vi "saveBackgroundMedian.vi"() -> ()   [LabVIEW 2012]
uses:
  <vilib>/userdefined/High Color/IMAQdx.ctl
  <vilib>/vision/driver/NI_Vision_Acquisition_Software.lvlib
  <vilib>/vision/NI_Vision_Development_Module.lvlib
  <resource>/objmgr/IMAQImage.rc
panel:
  out "element 2":i32
  out "element":i32
  out "Array":u8[][][](array[numeric])
  in  "Camera Name":T1
  out "Image Array":T2[](array[plugin-control])
  in  "Number of Images":i32=5
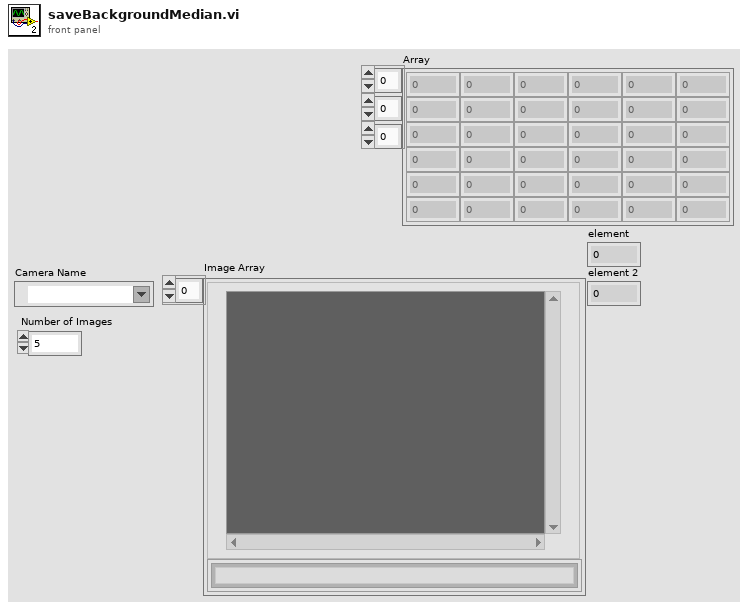
[diagram p1: front panel]
types:
  T1 = typedef "IMAQdx.ctl" = refnum<k21>
  T2 = typedef "IMAQ Image.ctl" = refnum<image>
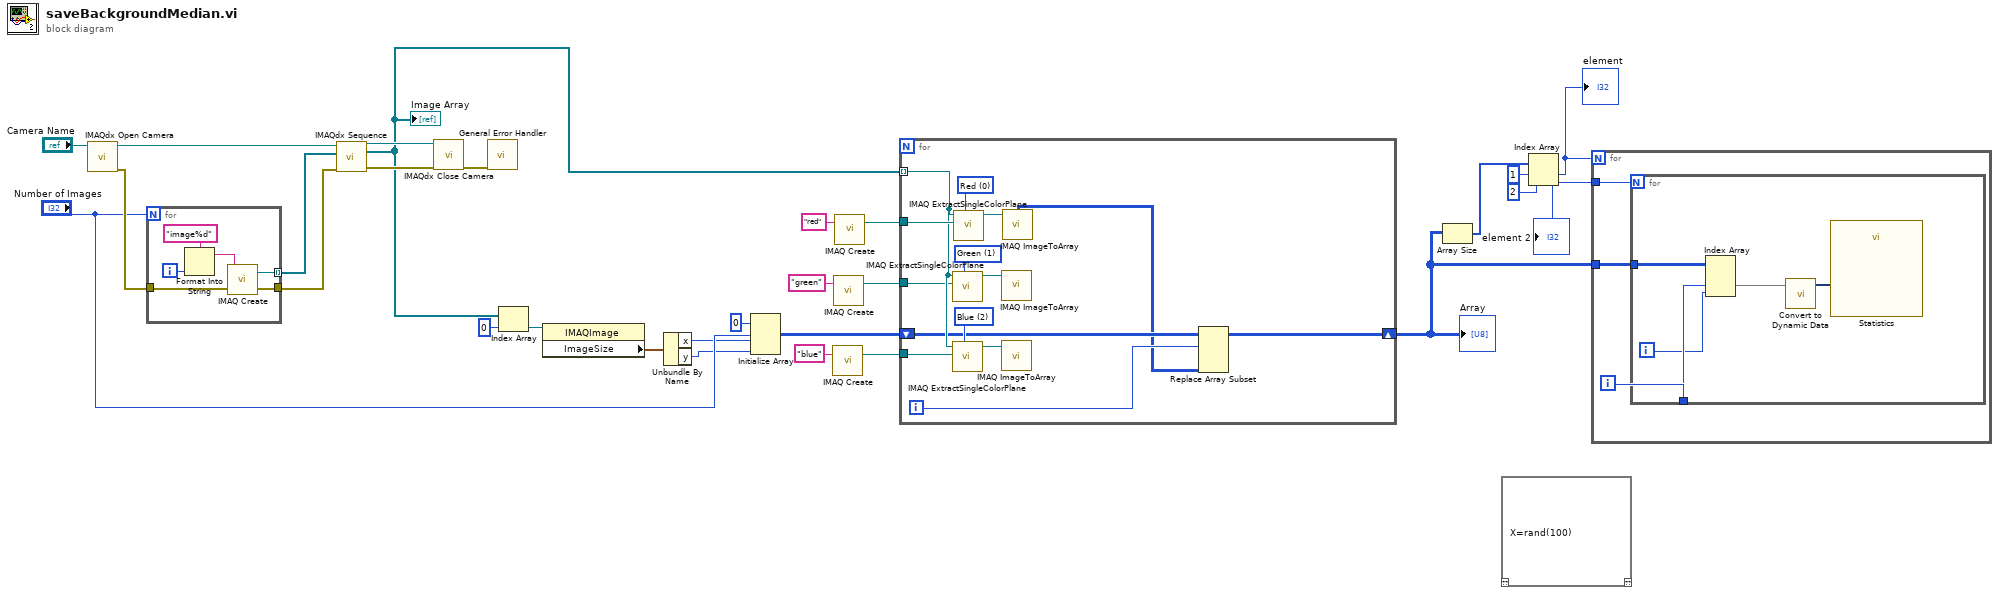
[diagram p0: block diagram]
diagram:
  n1 = call <vilib>:"IMAQdx Open Camera.vi"("Session In"="Camera Name") -> ("error out"=w27:errorcluster, "Session Out"=w23:T1)  [unwired: 2 in, 7 out]
  n2 = for {
    N: "Number of Images" -> [_]
    tunnel: w27 -> [w35]
    tunnel: [w34] -> w25 mode=indexing
    tunnel: [w33] -> w26
    i -> [w32]
    n3 = Format Into String(format string="image%d" ("Image Name"), w32) -> (resulting string=w31:string)  [unwired: 2 in, 1 out]
    n4 = call "IMAQ Create"("Image Name"=w31, "error in (no error)"=w35) -> ("New Image"=w34:T2, "error out"=w33:errorcluster)  [unwired: 2 in, 1 out]
  }
  n5 = call <vilib>:"IMAQdx Sequence.vi"("error in"=w26, "Images In"=w25, "Session In"=w23) -> ("error out"=w24:errorcluster, "Images Out"=w10:T2[], "Session Out"=w22:T1)  [unwired: 6 out]
  "Image Array" <- w10
  n6 = call <vilib>:"IMAQdx Close Camera.vi"("error in"=w24, "Session In"=w22) -> ("error out"=w28:errorcluster)  [unwired: 9 out]
  n7 = call <vilib>:"General Error Handler.vi"("error in (no error)"=w28) -> ()  [unwired: 1 in, 14 out]
  n8 = Index Array(array=w10, index=0) -> (element=w11:T2)
  n9 = property class="IMAQImage"(reference=w11) -> ("ImageSize"=w12:cluster{"x":i32, "y":i32})  [unwired: 1 in, 2 out]
  n10 = Unbundle By Name(w12) -> ("x"=w8:i32, "y"=w7:i32)
  n11 = Initialize Array(u8 0 ("element"), "Number of Images", w8, w7) -> (w14:u8[][][])
  n12 = call "IMAQ Create"("Image Name"="blue") -> ("New Image"=w16:T2)  [unwired: 3 in, 2 out]
  n13 = call "IMAQ Create"("Image Name"="green") -> ("New Image"=w17:T2)  [unwired: 3 in, 2 out]
  n14 = call "IMAQ Create"("Image Name"="red") -> ("New Image"=w20:T2)  [unwired: 3 in, 2 out]
  n15 = for {
    tunnel: w10 -> [w42] mode=indexing
    tunnel: w20 -> [w49]
    tunnel: w17 -> [w41]
    tunnel: w16 -> [w40]
    shift-right: [w37] -> w1
    shift-left: w14 -> [w39]
    i -> [w38]
    w43 = 2 items=["Red", "Green", "Blue", "Hue", "Saturation", "Luminance", "Value", "Intensity"] ("Color Plane")
    w44 = 1 items=["Red", "Green", "Blue", "Hue", "Saturation", "Luminance", "Value", "Intensity"] ("Color Plane")
    w45 = 0 items=["Red", "Green", "Blue", "Hue", "Saturation", "Luminance", "Value", "Intensity"] ("Color Plane")
    n16 = call "IMAQ ExtractSingleColorPlane"("Color Plane"=w44, "Image Dst"=w41, "Image Src"=w42) -> ("Image Dst Out"=w46:T2)  [unwired: 7 in, 1 out]
    n17 = call "IMAQ ExtractSingleColorPlane"("Color Plane"=w43, "Image Dst"=w40, "Image Src"=w42) -> ("Image Dst Out"=w47:T2)  [unwired: 7 in, 1 out]
    n18 = call "IMAQ ExtractSingleColorPlane"("Color Plane"=w45, "Image Dst"=w49, "Image Src"=w42) -> ("Image Dst Out"=w48:T2)  [unwired: 7 in, 1 out]
    n19 = call "IMAQ ImageToArray"("Image"=w46) -> ()  [unwired: 3 in, 5 out]
    n20 = call "IMAQ ImageToArray"("Image"=w47) -> ()  [unwired: 3 in, 5 out]
    n21 = call "IMAQ ImageToArray"("Image"=w48) -> ("Image Pixels (U8)"=w36:u8[][])  [unwired: 3 in, 4 out]
    n22 = Replace Array Subset(array=w39, new element=w36, index (dim 0)=w38) -> (w37:u8[][][])  [unwired: 2 in]
  }
  "Array" <- w1
  n23 = Array Size(array=w1) -> (size(s)=w6:i32[])
  n24 = script code="X=rand(100)"() -> ()  [unwired: 1 in, 1 out]
  n25 = Index Array(array=w6, index #1=1 ("index"), index #2=2 ("index")) -> (element #1=w4:i32, element #2=w2:i32)
  "element" <- w4
  "element 2" <- w2
  n26 = for {
    N: w4 -> [_]
    tunnel: w2 -> [w52]
    tunnel: w1 -> [w51]
    i -> [w50]
    n27 = for {
      N: w52 -> [_]
      tunnel: w51 -> [w57]
      tunnel: w50 -> [w56]
      i -> [w55]
      n28 = Index Array(array=w57, index (dim 1)=w56, index (dim 2)=w55) -> (element=w54:u8[])  [unwired: 1 in]
      n29 = call "Convert to Dynamic Data"("Array"=w54) -> ("Dynamic Data Type"=w53:dynamicdata)  [unwired: 3 in]
      n30 = call "Statistics"("Signals"=w53) -> ()  [unwired: 25 in, 2 out]
    }
  }
